vi "Give time find value for 1D data.vi"(9 "Time (lookup)":dbl, 10 "Data":dbl[](array[numeric]), 11 "Time (s)":dbl[](array[numeric])) -> (2 "data":dbl, 3 "time":dbl)   [LabVIEW 2021, in "RocketPlot.lvlib"]
uses:
  RocketPlot.lvlib
  <vilib>/gmath/NI_Gmath.lvlib
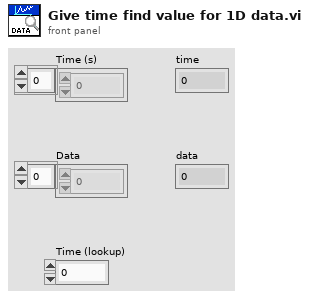
[diagram p1: front panel]
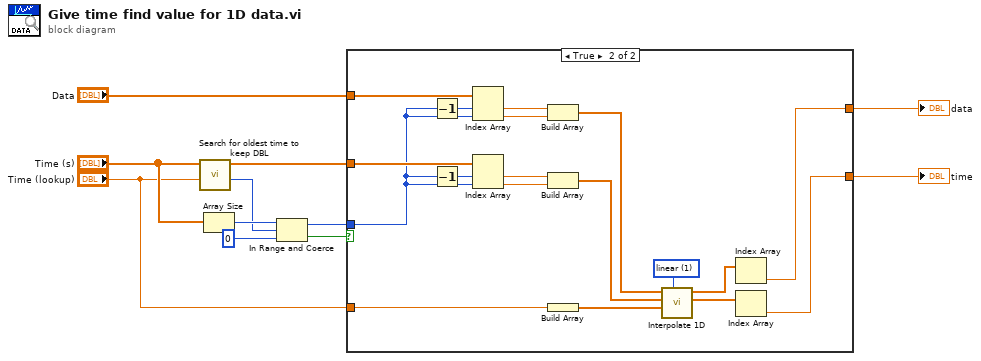
[diagram p0: block diagram]
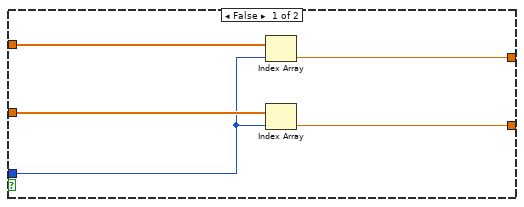
[diagram p2: hidden frame]
diagram:
  n1 = call "Search for oldest time to keep DBL.vi"("oldest time to keep"="Time (lookup)", "timestamps (incrementing)"="Time (s)") -> ("split index"=w1:i32, "timestamps (dup)"=w2:dbl[])  [unwired: 8 in]
  n2 = Array Size(array="Time (s)") -> (size(s)=w8:i32)
  n3 = In Range and Coerce(upper limit=w8, x=w1, lower limit=0) -> (coerced(x)=w6:i32, In Range?=w5:bool)
  n4 = case shown="True" w5 {
    tunnel: "Data" -> [w16 w34]
    tunnel: [w15 w18] -> w10
    tunnel: [w14 w17] -> w9
    tunnel: w2 -> [w13 w31]
    tunnel: w6 -> [w12 w30]
    tunnel: "Time (lookup)" -> [_ w23]
    frame False {
      n5 = Index Array(array=w16, index=w12) -> (element=w15:dbl)
      n6 = Index Array(array=w13, index=w12) -> (element=w14:dbl)
    }
    frame True {
      w21 = 1 items=["nearest", "linear", "spline", "cubic Hermite", "Lagrange"] ("method")
      n7 = Decrement(x=w30) -> (x-1=w33:i32)
      n8 = Decrement(x=w30) -> (x-1=w32:i32)
      n9 = Index Array(array=w34, index #1=w33, index #2=w30) -> (element #1=w29:dbl, element #2=w28:dbl)
      n10 = Index Array(array=w31, index #1=w32, index #2=w30) -> (element #1=w27:dbl, element #2=w26:dbl)
      n11 = Build Array(w29, w28) -> (w24:dbl[])
      n12 = Build Array(w27, w26) -> (w25:dbl[])
      n13 = Build Array(w23) -> (w22:dbl[])
      n14 = call <vilib>:"Interpolate 1D.vi"("method"=w21, "xi"=w22, "X"=w25, "Y"=w24) -> ("xi used"=w19:dbl[], "yi"=w20:dbl[])  [unwired: 5 in, 1 out]
      n15 = Index Array(array=w20) -> (element=w18:dbl)  [unwired: 1 in]
      n16 = Index Array(array=w19) -> (element=w17:dbl)  [unwired: 1 in]
    }
  }
  "data" <- w10
  "time" <- w9
